vi "Get Tree Items.vi"(8 "error in (no error)":errorcluster, 10 "Filter":T1, 11 "Result Model In":refnum<class "Result Model.lvclass">) -> (0 "error out":errorcluster, 2 "Tree Items":T2(array[cluster]))   [LabVIEW 2020, in "Result Model.lvclass"]
uses:
  Result Model.lvclass
  Tree Item Filter.ctl
  Result Model.lvclass/Result Model.ctl
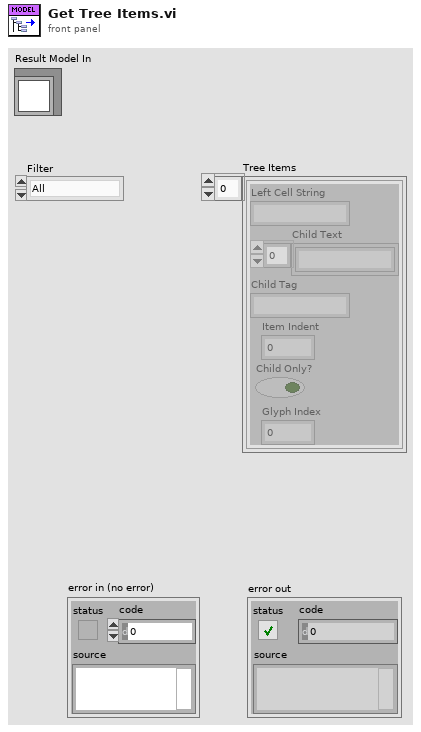
[diagram p1: front panel]
types:
  T1 = typedef "Result Model.lvclass/Tree Item Filter.ctl" = enum16{"All", "Only Fails", "Fails or else Not Executed"}
  T2 = cluster{"Left Cell String":string, "Child Text":string[], "Child Tag":string, "Item Indent":i32, "Child Only?":bool, "Glyph Index":i32}[]
  T3 = typedef "Result.lvlib/Status.ctl" = enum16{"", "Passed", "Failed", "Error", "Skipped", "Setup Error", "Broken", "Teardown Error"}
  T4 = cluster{"Left Cell String":string, "Child Text":string[], "Child Tag":string, "Item Indent":i32, "Child Only?":bool, "Glyph Index":i32}
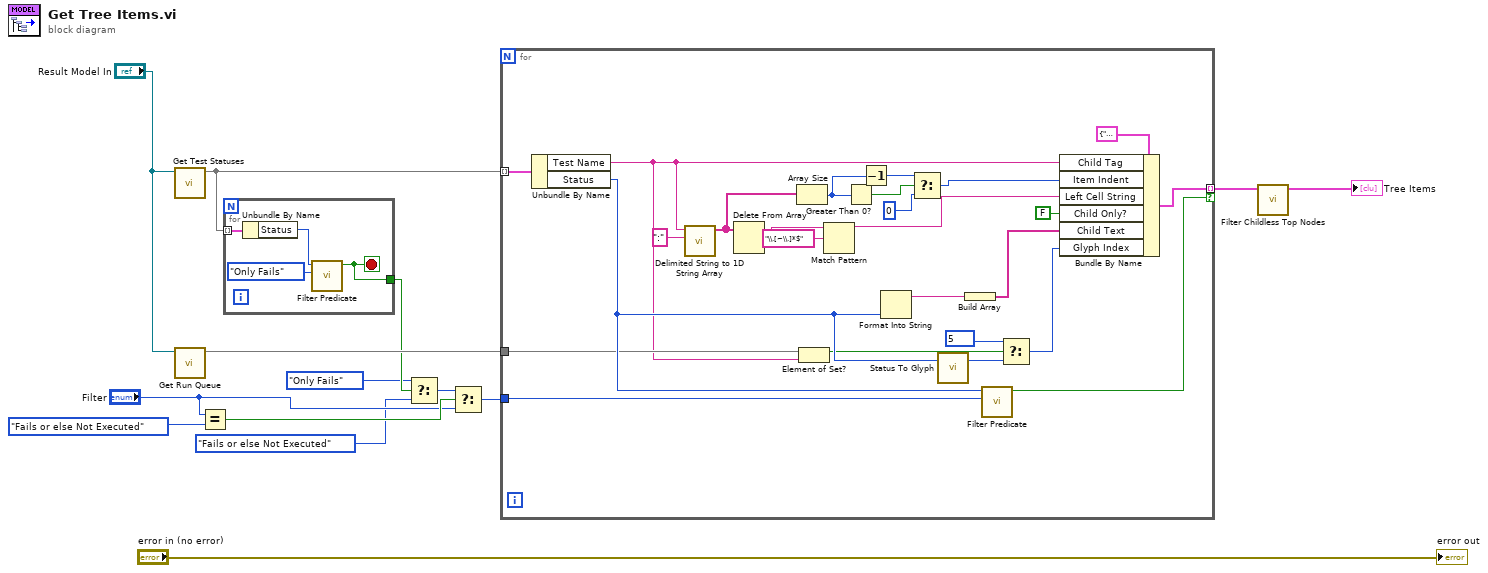
[diagram p0: block diagram]
diagram:
  n1 = call "Get Test Statuses.vi"("Result Model In"="Result Model In") -> ("Test Statuses"=w9:map{string, T3})  [unwired: 10 in]
  n2 = call "Get Run Queue.vi"("Result Model In"="Result Model In") -> ("Run Queue"=w12:set{string})  [unwired: 10 in]
  n3 = Equal?(x="Filter", y=Tree_Item_Filter."Fails or else Not Executed") -> (x = y?=w6:bool)
  n4 = for {
    tunnel: w9 -> [w18] mode=indexing
    tunnel: [w15] -> w4
    stop <- w15 stop-if-true
    n5 = Unbundle By Name(w18) -> ("Status"=w16:T3)
    n6 = call "Filter Predicate.vi"("Filter"=Tree_Item_Filter."Only Fails", "Status"=w16) -> ("Include?"=w15:bool)  [unwired: 9 in]
  }
  n7 = Select(t=Tree_Item_Filter."Only Fails" ("Filter"), s=w4, f=Tree_Item_Filter."Fails or else Not Executed" ("y")) -> (s? t:f=w1:T1)
  n8 = Select(t=w1, s=w6, f="Filter") -> (s? t:f=w8:T1)
  n9 = for {
    tunnel: w9 -> [w42] mode=indexing
    tunnel: [w41] -> w14 mode=indexing if=w27
    tunnel: w12 -> [w33]
    tunnel: w8 -> [w28]
    n10 = Unbundle By Name(w42) -> ("Test Name"=w21:string, "Status"=w36:T3)
    n11 = call <vilib>:"Delimited String to 1D String Array.vi"("delimiter"=":", "delimited string"=w21) -> ("string array"=w37:string[])  [unwired: 9 in]
    n12 = Delete From Array(array=w37) -> (deleted portion=w20:string)  [unwired: 2 in, 1 out]
    n13 = Array Size(array=w37) -> (size(s)=w25:i32)
    n14 = Element of Set?(10:w21, 11:w33) -> (3:w32:bool)
    n15 = Match Pattern(string=w20, regular expression="\\.[~\\.]*$") -> (before substring=w38:string)  [unwired: 1 in, 3 out]
    n16 = Greater Than 0?(x=w25) -> (x > 0?=w26:bool)
    n17 = Decrement(x=w25) -> (x-1=w24:i32)
    n18 = Format Into String(w36) -> (resulting string=w35:string)  [unwired: 3 in, 1 out]
    n19 = Select(t=w24, s=w26, f=0) -> (s? t:f=w23:i32)
    n20 = call "Status To Glyph.vi"("Status"=w36) -> ("Listbox Symbol Ring Constant"=w29:i32)  [unwired: 2 in]
    n21 = Build Array(w35) -> (w34:string[])
    n22 = call "Filter Predicate.vi"("Filter"=w28, "Status"=w36) -> ("Include?"=w27:bool)  [unwired: 9 in]
    n23 = Select(t=5 ("Listbox Symbol Ring Constant"), s=w32, f=w29) -> (s? t:f=w30:i32)
    n24 = Bundle By Name(cluster=T4 {"Left Cell String"="", "Child Text"=[], "Child Tag"="", "Item Indent"=0, "Child Only?"=FALSE, "Glyph Index"=0} ("Item"), "Child Tag"=w21, "Item Indent"=w23, "Left Cell String"=w38, "Child Only?"=FALSE, "Child Text"=w34, "Glyph Index"=w30) -> (w41:T4)
  }
  n25 = call "Filter Childless Top Nodes.vi"("All Items"=w14) -> ("Filtered Items"=→"Tree Items":T2)  [unwired: 10 in]
  "error out" <- "error in (no error)"
